vi "Load RC Config From File.vi"(8 "Error In":errorcluster, 11 "Aircraft ID":u8) -> (0 "Error Out":errorcluster)   [LabVIEW 2014]
uses:
  Controls/Aircraft RC Data.ctl
  <vilib>/Utility/xml.llb/Read From XML File(array).vi
  Set Aircraft RC.vi
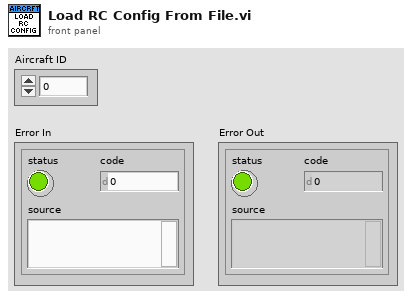
[diagram p1: front panel]
types:
  T1 = typedef "Aircraft RC Data.ctl" = cluster{"Channel 1 Min":i16, "Channel 1 Max":i16, "Channel 2 Min":i16, "Channel 2 Max":i16, "Channel 3 Min":i16, "Channel 3 Max":i16, "Channel 4 Min":i16, "Channel 4 Max":i16}
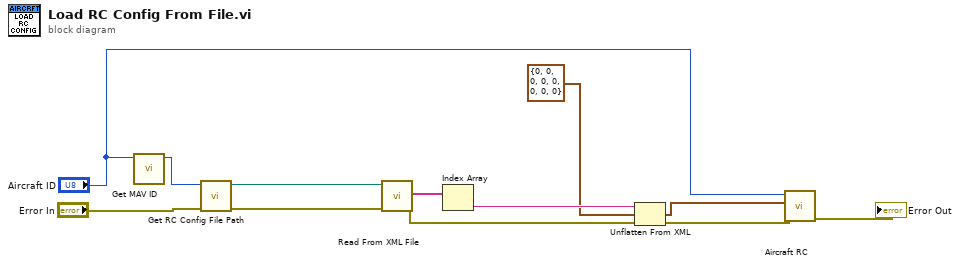
[diagram p0: block diagram]
diagram:
  n1 = call "Get MAV ID.vi"("Aircraft Index"="Aircraft ID") -> ("Aircraft ID"=w1:u8)  [unwired: 9 in, 1 out]
  n2 = call "Get RC Config File Path.vi"("Error In"="Error In", "Aircraft ID"=w1) -> ("Error Out"=w9:errorcluster, "Anchor Config File Path"=w10:path)  [unwired: 8 in]
  n3 = call-poly <vilib>:"Read From XML File.vi"("error in (no error)"=w9, "XML File Path"=w10) -> ("error out"=w6:errorcluster, "XML Elements"=w12:string[])  [unwired: 7 in, 1 out]
  n4 = Index Array(array=w12) -> (element=w11:string)  [unwired: 1 in]
  n5 = Unflatten From XML(xml string=w11, type=T1 {"Channel 1 Min"=0, "Channel 1 Max"=0, "Channel 2 Min"=0, "Channel 2 Max"=0, "Channel 3 Min"=0, "Channel 3 Max"=0, "Channel 4 Min"=0, "Channel 4 Max"=0} ("Aircraft RC Data"), error in (no error)=w6) -> (value=w4:T1, error out=w5:errorcluster)
  n6 = call-poly "Aircraft RC.vi"("Error In"=w5, "Aircraft RC Data"=w4, "Aircraft ID"="Aircraft ID") -> ("Error Out"=→"Error Out":errorcluster)  [unwired: 8 in]
